vi "BIO_write_filename.vi"(8 "error in (no error)":errorcluster, 10 "File path":string, 11 "BIO in":refnum<class "BIO.lvclass">) -> (0 "error out":errorcluster, 3 "BIO out":refnum<class "BIO.lvclass">)   [LabVIEW 2013, in "OpenSSL Socket.lvlib" / "BIO.lvclass"]
uses:
  BIO.lvclass
  SSL-Lib/SSL-Lib.lvclass/SSL-Lib.ctl
  BIO.lvclass/BIO.ctl
  SSL-Lib/Read Crypto Library Path.vi
  Read Handle.vi
  SSL-Lib/SSL-Lib.lvclass
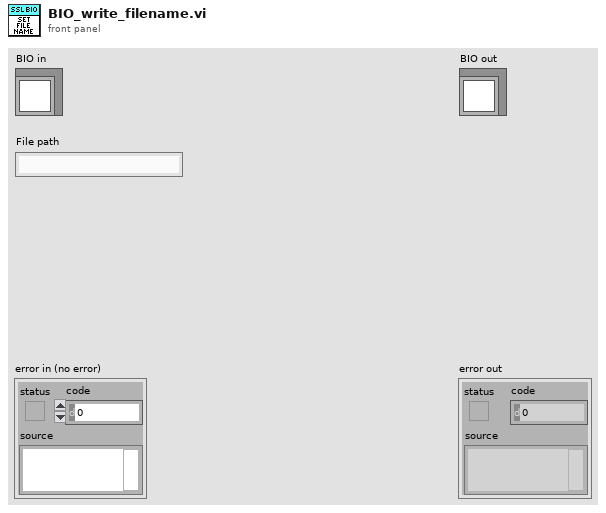
[diagram p1: front panel]
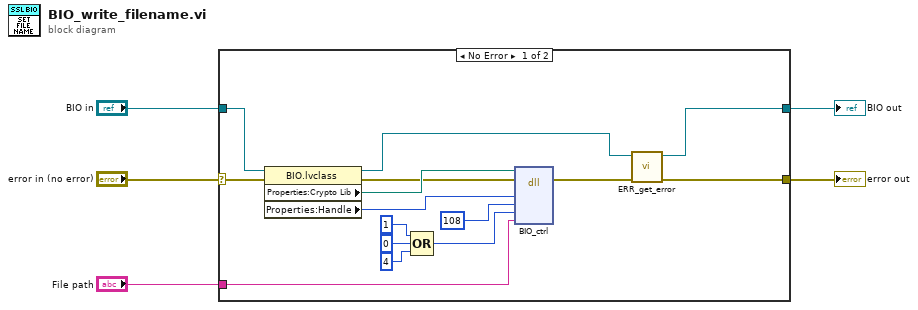
[diagram p0: block diagram]
diagram:
  n1 = case shown="No Error" "error in (no error)" {
    selector: "error in (no error)" -> [w18 w22]
    tunnel: [w12 w22] -> w4
    tunnel: [w10 w21] -> w2
    tunnel: "BIO in" -> [w17 w21]
    tunnel: "File path" -> [w19 _]
    frame No Error {
      n2 = property class="BIO.lvclass"(reference=w17, error in=w18) -> (reference out=w11:refnum<class "BIO.lvclass">, error out=w14:errorcluster, "Properties:Crypto Lib"=w15:path, "Properties:Handle"=w16:u64)
      n3 = Compound Arithmetic op=OR(1 ("larg"), 0 ("y"), 4 ("y")) -> (w8:i32)
      n4 = dll-call lib="C:/Program Files (x86)/National Instruments/Shared/nissl/NIlibeay32.dll" fn="BIO_ctrl"(path in=w15, error in=w14, "BIO"=w16, "cmd"=108, "larg"=w8, "parg"=w19) -> (error out=w13:errorcluster)  [unwired: 6 in, 1 out]
      n5 = call "ERR_get_error.vi"("error in (no error)"=w13, "SSL-Lib in"=w11) -> ("error out"=w12:errorcluster, "SSL-Lib out"=w10:refnum<class "BIO.lvclass">)  [unwired: 8 in]
    }
    frame Error {
    }
  }
  "error out" <- w4
  "BIO out" <- w2
